vi "Neural Network.vi"(1 "Weights, W":dbl[][](array[numeric]) format="%.3f", 2 "Function, y":dbl[](array[numeric]) format="%.3f", 3 "Control, U":ext=1.0) -> (0 "Outputs, z":dbl[](array[numeric]) format="%.3f")   [LabVIEW 2022 SP3]
uses:
  <vilib>/Analysis/baseanly.llb/Vector x A.vi
  <vilib>/Analysis/NI_AALBase.lvlib
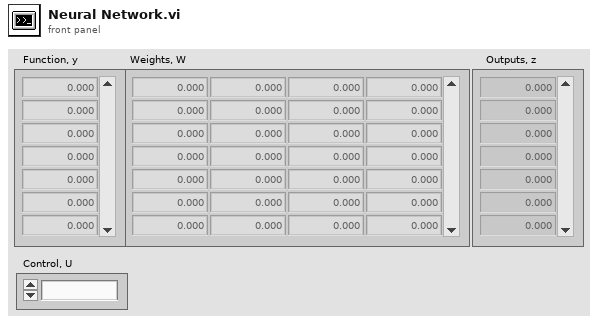
[diagram p1: front panel]
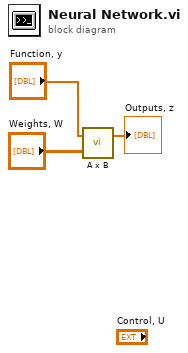
[diagram p0: block diagram]
diagram:
  n1 = call-poly <vilib>:"A x B.vi"("Matrix A"="Weights, W", "Vector V'"="Function, y") -> ("V' x A"=→"Outputs, z":dbl[])  [unwired: 1 out]
